vi "RSZVB Set Meas Bandwidth Selectivity.vi"(8 "error in (no error)":errorcluster {"code" format="%.0x"}, 9 "Meas Bandwidth Selectivity (0: Normal)":i32(ring) items=["Normal", "High"], 10 "Channel (1)":i32=1, 11 "VISA session":refnum<visa-resource-name>) -> (0 "error out":errorcluster {"code" format="%.0x"}, 3 "dup VISA session":refnum<visa-resource-name>)   [LabVIEW 2011]
doc: "This VI defines the selectivity of the IF filter for an unsegmented sweep. The value is also used for all segments of a segmented sweep, provided that separate selectivity setting is disabled ([SENSe<Ch>:]SEGMent<Seg>:BWIDth[:RESolution]:CONTrol OFF). \n\nNote(s):\n\n(1) This VI can be used only with R&S ZVA and R&S ZVT instruments.\n\nRemote-control command(s):\n[SENSe<Ch>:]BANDwidth|BWIDth[:RESolution]:SELect NORMal | HIGH"
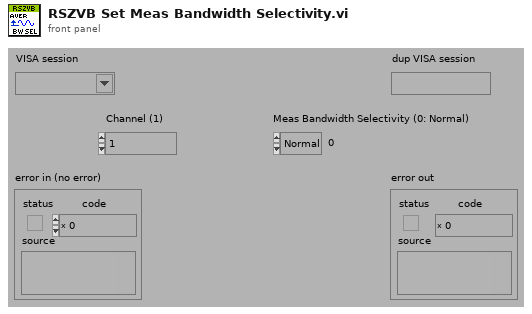
[diagram p1: front panel]
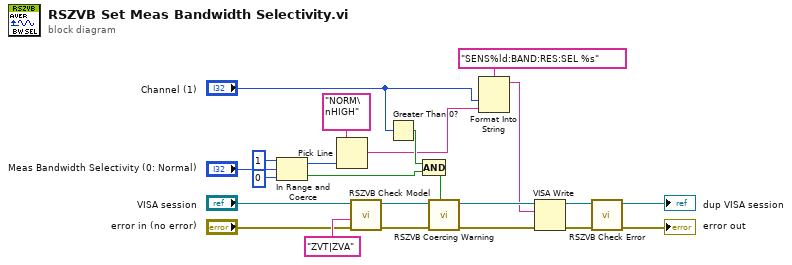
[diagram p0: block diagram]
diagram:
  n1 = In Range and Coerce(upper limit=1, x="Meas Bandwidth Selectivity (0: Normal)", lower limit=0) -> (coerced(x)=w5:i32, In Range?=w3:bool)
  n2 = Pick Line(multi-line string="NORM\nHIGH", line index=w5) -> (output string=w4:string)  [unwired: 1 in]
  n3 = call "RSZVB Check Model.vi"("error in (no error)"="error in (no error)", "Model"="ZVT|ZVA" ("Options"), "VISA session"="VISA session") -> ("error out"=w15:errorcluster, "dup VISA session"=w14:refnum<visa-resource-name>)  [unwired: 7 in]
  n4 = Greater Than 0?(x="Channel (1)") -> (x > 0?=w16:bool)
  n5 = Compound Arithmetic op=AND(w16, w3) -> (w18:bool)
  n6 = call "RSZVB Coercing Warning.vi"("In Range?"=w18, "error in (no error)"=w15, "VISA session"=w14) -> ("error out"=w21:errorcluster, "dup VISA session"=w22:refnum<visa-resource-name>)  [unwired: 7 in]
  n7 = Format Into String(format string="SENS%ld:BAND:RES:SEL %s", "Channel (1)", w4) -> (resulting string=w17:string)  [unwired: 2 in, 1 out]
  n8 = VISA Write(VISA resource name=w22, write buffer=w17, error in (no error)=w21) -> (VISA resource name out=w19:refnum<visa-resource-name>, error out=w20:errorcluster)  [unwired: 1 out]
  n9 = call "RSZVB Check Error.vi"("error in (no error)"=w20, "VISA session"=w19) -> ("error out"=→"error out":errorcluster, "dup VISA session"=→"dup VISA session":refnum<visa-resource-name>)  [unwired: 8 in]
